vi "Switch Protection Signal.vi"(8 "error in (no error)":errorcluster, 9 "Signal Page GUID":string, 10 "Protection Value GUID":string, 11 "Node Ptr":T1 format="%.0x") -> (0 "error out":errorcluster)   [LabVIEW 2015, in "Protection and Counter Support System Explorer.lvlib"]
uses:
  Protection and Counter Support System Explorer.lvlib
  <vilib>/NI Veristand/Custom Device API/Custom Device Item Ref.ctl
  <vilib>/NI Veristand/Custom Device API/Custom Device Channel Type.ctl
  Shared/Properties Lookup.vi
  <vilib>/NI Veristand/Custom Device API/Get Item Property (String Array).vi
  <vilib>/NI VeriStand/Custom Device API/Custom Device API.lvlib
  <vilib>/NI VeriStand/Custom Device Tools/Custom Device Utility Library/Custom Device Utility Library.lvlib
  Shared/Protection and Counter Support Shared.lvlib
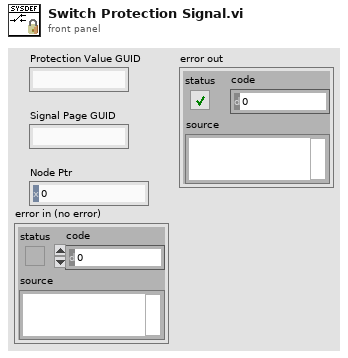
[diagram p1: front panel]
types:
  T1 = typedef "Custom Device API.lvlib/Custom Device Item Ref.ctl" = u64
  T2 = typedef "Custom Device API.lvlib/Custom Device Channel Type.ctl" = enum16{"Input", "Output"}
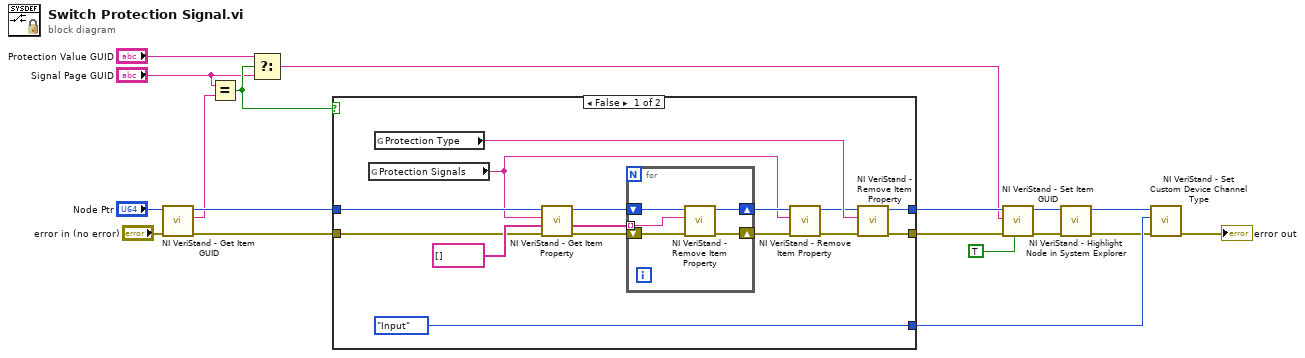
[diagram p0: block diagram]
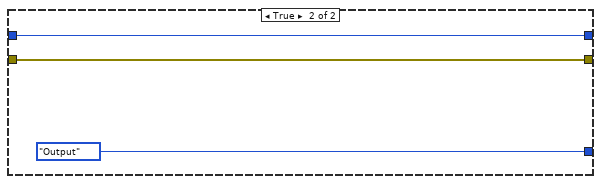
[diagram p2: hidden frame]
diagram:
  n1 = call <vilib>:"NI VeriStand - Get Item GUID.vi"("error in (no error)"="error in (no error)", "Item Ref in"="Node Ptr") -> ("error out"=w10:errorcluster, "GUID"=w3:string, "Item Ref out"=w12:T1)  [unwired: 7 in]
  n2 = Equal?(x="Signal Page GUID", y=w3) -> (x = y?=w14:bool)
  n3 = Select(t="Protection Value GUID", s=w14, f="Signal Page GUID") -> (s? t:f=w5:string)
  n4 = case shown="False" w14 {
    tunnel: w10 -> [w23 w39]
    tunnel: [w22 w39] -> w11
    tunnel: w12 -> [w20 w40]
    tunnel: [w21 w40] -> w13
    tunnel: [Custom_Device_Channel_Type."Input" ("Type") Custom_Device_Channel_Type."Output" ("Type")] -> w18
    frame False {
      n5 = global read "Properties Lookup.vi" "Protection Signals"() -> (w19:string)
      n6 = global read "Properties Lookup.vi" "Protection Type"() -> (w26:string)
      n7 = call-poly <vilib>:"NI VeriStand - Get Item Property.vi"("error in (no error)"=w23, "Default Value"=string[] [], "Property Name"=w19, "Item Ref in"=w20) -> ("error out"=w30:errorcluster, "Value"=w28:string[], "Item Ref out"=w29:T1)  [unwired: 4 in, 1 out]
      n8 = for {
        shift-right: [w33] -> w25
        shift-left: w29 -> [w37]
        tunnel: w28 -> [w35] mode=indexing
        shift-right: [w34] -> w27
        shift-left: w30 -> [w36]
        n9 = call <vilib>:"NI VeriStand - Remove Item Property.vi"("error in (no error)"=w36, "Property Name"=w35, "Item Ref in"=w37) -> ("error out"=w34:errorcluster, "Item Ref out"=w33:T1)  [unwired: 6 in, 1 out]
      }
      n10 = call <vilib>:"NI VeriStand - Remove Item Property.vi"("Property Name"=w19, "Item Ref in"=w25) -> ("Item Ref out"=w24:T1)  [unwired: 7 in, 2 out]
      n11 = call <vilib>:"NI VeriStand - Remove Item Property.vi"("error in (no error)"=w27, "Property Name"=w26, "Item Ref in"=w24) -> ("error out"=w22:errorcluster, "Item Ref out"=w21:T1)  [unwired: 6 in, 1 out]
    }
    frame True {
    }
  }
  n12 = call <vilib>:"NI VeriStand - Set Item GUID.vi"("Refresh System Explorer Tree? (F)"=TRUE, "error in (no error)"=w11, "GUID"=w5, "Item Ref in"=w13) -> ("error out"=w9:errorcluster, "Item Ref out"=w8:T1)  [unwired: 6 in]
  n13 = call <vilib>:"NI VeriStand - Highlight Node in System Explorer.vi"("error in (no error)"=w9, "Item Ref in"=w8) -> ("error out"=w16:errorcluster, "Node Ptr dup"=w15:T1)  [unwired: 8 in]
  n14 = call <vilib>:"NI VeriStand - Set Custom Device Channel Type.vi"("error in (no error)"=w16, "Type"=w18, "Channel Ref in"=w15) -> ("error out"=→"error out":errorcluster)  [unwired: 7 in, 1 out]
